vi "libtiff3 write StripedPage raw U16-mod.vi"(7 "totalpages":i32, 8 "error in (no error)":errorcluster, 9 "page":u32, 10 "Image":T1, 11 "Handle":i32) -> (0 "error out":errorcluster, 3 "Handle out":i32)   [LabVIEW 2017]
doc: "SciScan 1.0 151216\nWrite a U16 page using LIBTIFFwriteRawStrip to a file previously open for writing"
uses:
  <vilib>/vision/Image Controls.llb/IMAQ Image.ctl
  DLLs/libtiff3 (32).dll
panel:
  in  "Image Pixels (U16)":u16[][](array[numeric])
  out "status_compression":i32
  out "status width":i32
  out "status_length":i32
  out "status_spp":i32
  out "status_bps":i32
  out "status_orientation":i32
  out "status_planarconfig":i32
  out "status_photo":i32
  out "status_rowperstrip":i32
  out "status_writerawstrip":i32
  out "status_subfile":i32
  out "status_writedir":i32
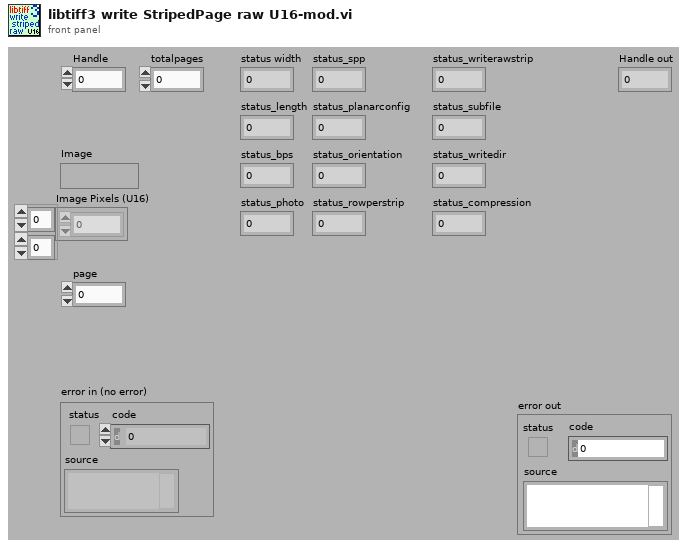
[diagram p1: front panel]
types:
  T1 = typedef "IMAQ Image.ctl" = refnum<image>
  T2 = cluster{"LastStripSize in bytes":i32, "LastStripRows":i32, "Last sripSize in pixels":i32}
  T3 = cluster{"StripSize in bytes":i32, "RowsPerStrip":u32, "StripSize in pixels":i32}
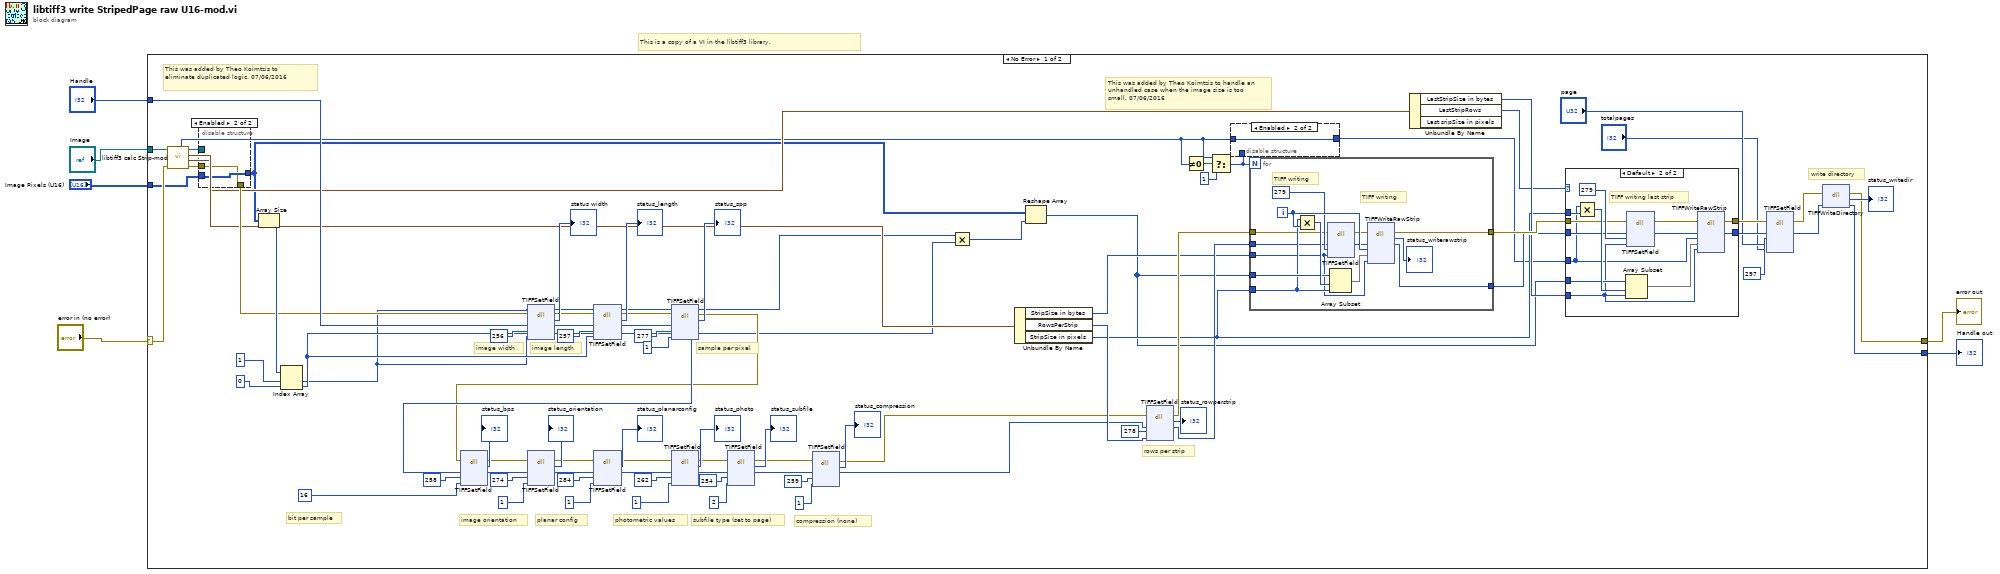
[diagram p0: block diagram]
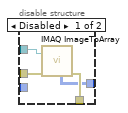
[diagram p3: hidden frame]
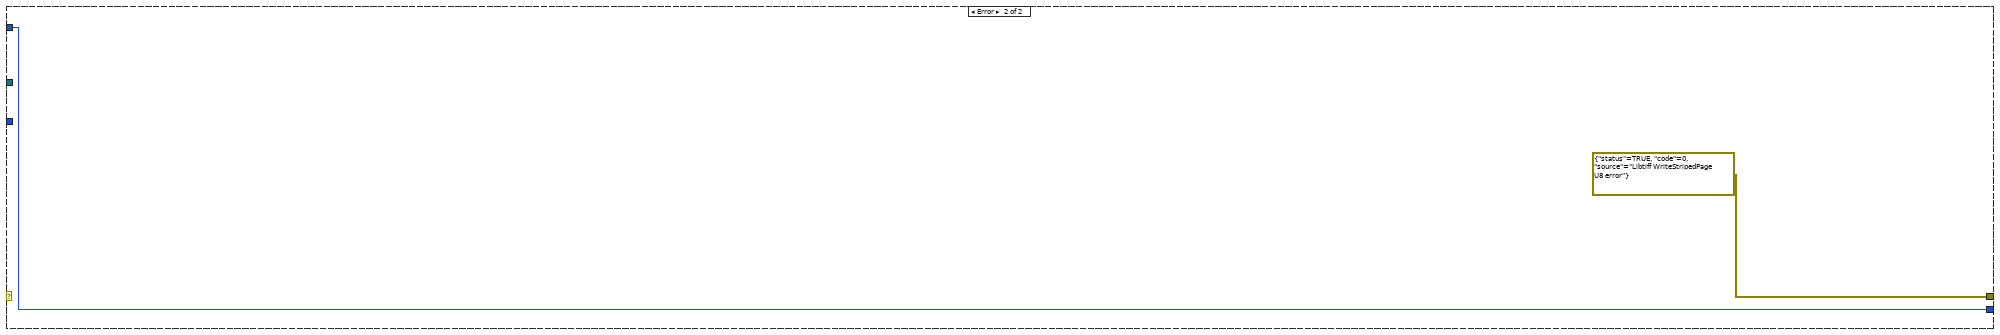
[diagram p5: hidden frame]
diagram:
  # "This is a copy of a VI in the libtiff3 library."
  n1 = case shown="No Error" "error in (no error)" {
    selector: "error in (no error)" -> [w30 _]
    tunnel: "Handle" -> [w63 w131]
    tunnel: [w59 w131] -> w5
    tunnel: [w8 errorcluster {"status"=TRUE, "code"=0, "source"="Libtiff WriteStripedPage U8 error"} ("error out")] -> w4
    tunnel: "Image" -> [w44 _]
    tunnel: "Image Pixels (U16)" -> [w15 _]
    frame No Error {
      # "This was added by Theo Koimtzis to eliminate duplicated logic. 07/06/2016"
      # "This was added by Theo Koimtzis to handle an unhandled case when the image size is too small. 07/06/2016"
      # "rows per strip"
      # "compression (none)"
      # "write directory"
      # "subfile type (set to page)"
      # "photometric values"
      # "planar config"
      # "image orientation"
      # "bit per sample"
      # "sample per pixel"
      # "image length"
      # "image width"
      n2 = call "libtiff3 calc Strip-mod.vi"("error in (no error)"=w30, "ImageIn"=w44) -> ("error out"=w43:errorcluster, "LastStrip"=w29:T2, "Strip"=w41:T3, "ImageOut"=w42:T1, "NumberOfStrips"=w12:i32)  [unwired: 5 in]
      n3 = disable-structure shown="Enabled" {
        disable-tunnel: [w112 w113] -> w54
        disable-tunnel: w43 -> [w111 w113]
        disable-tunnel: w42 -> [w110 _]
        disable-tunnel: [w109 w114] -> w25
        disable-tunnel: w15 -> [_ w114]
        frame Disabled {
          n4 = call "IMAQ ImageToArray"("error in (no error)"=w111, "Image"=w110) -> ("Image Pixels (U16)"=w109:u16[][], "error out"=w112:errorcluster)  [unwired: 1 in, 4 out]
        }
        frame Enabled {
        }
      }
      n5 = Array Size(array=w25) -> (size(s)=w60:i32[])
      n6 = Index Array(array=w60, index #1=1 ("index"), index #2=0 ("index")) -> (element #1=w39:i32, element #2=w40:i32)
      n7 = dll-call lib="C:/Users/ucbtspu/OneDrive - University College London/Local SCC/SilverLab-Microscope-R3-LV2013/support/Libtiff3/DLLs/libtiff3 (32).dll" fn="TIFFSetField"(error in=w54, "Handle"=w63, "TIFF_tag"=256, "Value"=w39) -> (error out=w53:errorcluster, "return type"=→"status width":i32, "Handle"=w90:i32)  [unwired: 4 in, 1 out]
      n8 = dll-call lib="C:/Users/ucbtspu/OneDrive - University College London/Local SCC/SilverLab-Microscope-R3-LV2013/support/Libtiff3/DLLs/libtiff3 (32).dll" fn="TIFFSetField"(error in=w53, "Handle"=w90, "TIFF_tag"=257, "value"=w40) -> (error out=w52:errorcluster, "return type"=→"status_length":i32, "Handle"=w87:i32)  [unwired: 4 in, 1 out]
      n9 = dll-call lib="C:/Users/ucbtspu/OneDrive - University College London/Local SCC/SilverLab-Microscope-R3-LV2013/support/Libtiff3/DLLs/libtiff3 (32).dll" fn="TIFFSetField"(error in=w52, "Handle"=w87, "TIFF_tag"=277, "value"=u32 1) -> (error out=w51:errorcluster, "return type"=→"status_spp":i32, "Handle"=w84:i32)  [unwired: 4 in, 1 out]
      n10 = dll-call lib="C:/Users/ucbtspu/OneDrive - University College London/Local SCC/SilverLab-Microscope-R3-LV2013/support/Libtiff3/DLLs/libtiff3 (32).dll" fn="TIFFSetField"(error in=w51, "Handle"=w84, "TIFF_tag"=258, "value"=u32 16) -> (error out=w50:errorcluster, "return type"=→"status_bps":i32, "Handle"=w81:i32)  [unwired: 4 in, 1 out]
      n11 = dll-call lib="C:/Users/ucbtspu/OneDrive - University College London/Local SCC/SilverLab-Microscope-R3-LV2013/support/Libtiff3/DLLs/libtiff3 (32).dll" fn="TIFFSetField"(error in=w50, "Handle"=w81, "TIFF_tag"=274, "value"=u32 1) -> (error out=w49:errorcluster, "return type"=→"status_orientation":i32, "Handle"=w77:i32)  [unwired: 4 in, 1 out]
      n12 = dll-call lib="C:/Users/ucbtspu/OneDrive - University College London/Local SCC/SilverLab-Microscope-R3-LV2013/support/Libtiff3/DLLs/libtiff3 (32).dll" fn="TIFFSetField"(error in=w49, "Handle"=w77, "TIFF_tag"=284, "value"=u32 1) -> (error out=w48:errorcluster, "return type"=→"status_planarconfig":i32, "Handle"=w73:i32)  [unwired: 4 in, 1 out]
      n13 = dll-call lib="C:/Users/ucbtspu/OneDrive - University College London/Local SCC/SilverLab-Microscope-R3-LV2013/support/Libtiff3/DLLs/libtiff3 (32).dll" fn="TIFFSetField"(error in=w48, "Handle"=w73, "TIFF_tag"=262, "value"=u32 1) -> (error out=w47:errorcluster, "return type"=→"status_photo":i32, "Handle"=w68:i32)  [unwired: 4 in, 1 out]
      n14 = dll-call lib="C:/Users/ucbtspu/OneDrive - University College London/Local SCC/SilverLab-Microscope-R3-LV2013/support/Libtiff3/DLLs/libtiff3 (32).dll" fn="TIFFSetField"(error in=w47, "Handle"=w68, "TIFF_tag"=254, "value"=u32 2) -> (error out=w46:errorcluster, "return type"=→"status_subfile":i32, "Handle"=w56:i32)  [unwired: 4 in, 1 out]
      n15 = dll-call lib="C:/Users/ucbtspu/OneDrive - University College London/Local SCC/SilverLab-Microscope-R3-LV2013/support/Libtiff3/DLLs/libtiff3 (32).dll" fn="TIFFSetField"(error in=w46, "Handle"=w56, "TIFF_tag"=259, "value"=u32 1) -> (error out=w32:errorcluster, "return type"=→"status_compression":i32, "Handle"=w31:i32)  [unwired: 4 in, 1 out]
      n16 = Multiply(x=w39, y=w40) -> (x*y=w38:i32)
      n17 = Unbundle By Name(w41) -> ("StripSize in bytes"=w24:i32, "RowsPerStrip"=w35:u32, "StripSize in pixels"=w23:i32)
      n18 = Reshape Array(w25, w38) -> (w7:u16[])
      n19 = dll-call lib="C:/Users/ucbtspu/OneDrive - University College London/Local SCC/SilverLab-Microscope-R3-LV2013/support/Libtiff3/DLLs/libtiff3 (32).dll" fn="TIFFSetField"(error in=w32, "Handle"=w31, "TIFF_tag"=278, "value"=w35) -> (error out=w33:errorcluster, "return type"=→"status_rowperstrip":i32, "Handle"=w34:i32)  [unwired: 4 in, 1 out]
      n20 = Not Equal To 0?(x=w12) -> (x != 0?=w14:bool)
      n21 = Select(t=w12, s=w14, f=1) -> (s? t:f=w11:i32)
      n22 = disable-structure shown="Enabled" {
        disable-tunnel: w12 -> [_ w94]
        disable-tunnel: [w93 w94] -> w10
        disable-tunnel: w11 -> [w93 _]
        frame Disabled {
        }
        frame Enabled {
        }
      }
      n23 = for {
        N: w11 -> [_]
        tunnel: [w107] -> w27
        tunnel: [w106] -> w28
        tunnel: w7 -> [w103]
        tunnel: w23 -> [w101]
        tunnel: w34 -> [w97]
        tunnel: w33 -> [w99]
        tunnel: w24 -> [w95]
        i -> [w105]
        # "TIFF writing"
        # "TIFF writing"
        n24 = Multiply(x=w101, y=w105) -> (x*y=w104:i32)
        n25 = dll-call lib="C:/Users/ucbtspu/OneDrive - University College London/Local SCC/SilverLab-Microscope-R3-LV2013/support/Libtiff3/DLLs/libtiff3 (32).dll" fn="TIFFSetField"(error in=w99, "Handle"=w97, "TIFF_tag"=279, "value"=w95) -> (error out=w98:errorcluster, "Handle"=w96:i32)  [unwired: 4 in, 2 out]
        n26 = Array Subset(array=w103, index=w104, length=w101) -> (w102:u16[])
        n27 = dll-call lib="C:/Users/ucbtspu/OneDrive - University College London/Local SCC/SilverLab-Microscope-R3-LV2013/support/Libtiff3/DLLs/libtiff3 (32).dll" fn="TIFFWriteRawStrip"(error in=w98, "Handle"=w96, "strip"=w105, "buffer"=w102, "length"=w95) -> (error out=w106:errorcluster, "return type"=→"status_writerawstrip":i32, "Handle"=w107:i32)  [unwired: 5 in, 1 out]
      }
      n28 = Unbundle By Name(w29) -> ("LastStripSize in bytes"=w26:i32, "LastStripRows"=w22:i32)  [unwired: 1 out]
      n29 = case shown="Default" w22 {
        tunnel: w28 -> [w116 w124]
        tunnel: w27 -> [w115 w123]
        tunnel: w7 -> [_ w122]
        tunnel: [w116 w121] -> w21
        tunnel: [w115 w120] -> w20
        tunnel: w26 -> [_ w119]
        tunnel: w23 -> [_ w118]
        tunnel: w10 -> [_ w117]
        frame 0 {
        }
        frame Default {
          # "TIFF writing last strip"
          n30 = Multiply(x=w117, y=w118) -> (x*y=w125:i32)
          n31 = Array Subset(array=w122, index=w125, length=w119) -> (w126:u16[])
          n32 = dll-call lib="C:/Users/ucbtspu/OneDrive - University College London/Local SCC/SilverLab-Microscope-R3-LV2013/support/Libtiff3/DLLs/libtiff3 (32).dll" fn="TIFFSetField"(error in=w124, "Handle"=w123, "TIFF_tag"=279, "value"=w119) -> (error out=w128:errorcluster, "Handle"=w129:i32)  [unwired: 4 in, 2 out]
          n33 = dll-call lib="C:/Users/ucbtspu/OneDrive - University College London/Local SCC/SilverLab-Microscope-R3-LV2013/support/Libtiff3/DLLs/libtiff3 (32).dll" fn="TIFFWriteRawStrip"(error in=w128, "Handle"=w129, "strip"=w117, "buffer"=w126, "length"=w119) -> (error out=w121:errorcluster, "Handle"=w120:i32)  [unwired: 5 in, 2 out]
        }
      }
      n34 = dll-call lib="C:/Users/ucbtspu/OneDrive - University College London/Local SCC/SilverLab-Microscope-R3-LV2013/support/Libtiff3/DLLs/libtiff3 (32).dll" fn="TIFFSetField"(error in=w21, "Handle"=w20, "TIFF_tag"=297, "page"="page", "totalpages"="totalpages") -> (error out=w9:errorcluster, "Handle"=w19:i32)  [unwired: 5 in, 2 out]
      n35 = dll-call lib="C:/Users/ucbtspu/OneDrive - University College London/Local SCC/SilverLab-Microscope-R3-LV2013/support/Libtiff3/DLLs/libtiff3 (32).dll" fn="TIFFWriteDirectory"(error in=w9, "Handle"=w19) -> (error out=w8:errorcluster, "return type"=→"status_writedir":i32, "Handle"=w59:i32)  [unwired: 2 in, 1 out]
    }
    frame Error {
    }
  }
  "Handle out" <- w5
  "error out" <- w4
